vi "Teleop.vi"(10 "Match Info":T1={"Autonomous Elapsed Seconds"=0.0, "TeleOp Elapsed Seconds"=0.0, "Disabled Elapsed Seconds"=0.0, "Visited Autonomous"=FALSE, "Visited TeleOp"=FALSE, "Visited Disabled"=FALSE, "Autonomous Settings"={"Autonomous Style"=enum."Independent", "VI Refnum"=refnum}}, 11 "Call Context":T2) -> ()   [LabVIEW 2016]
doc: "This VI is called for each TeleOp packet received from the DS where the robot is not disabled. It is often used to read from the joysticks and update I/O or to update setpoints for timed control loops. It should complete and return within 20 milliseconds or it may miss DS packets."
uses:
  <vilib>/Rock Robotics/WPI/DriverStation/WPI_DriverStationDerivedRobotMode.ctl
  <vilib>/Rock Robotics/WPI/DriverStation/WPI_DriverStationMatch Info.ctl
  <vilib>/Rock Robotics/WPI/Solenoid/WPI_SolenoidValue.ctl
  <vilib>/Rock Robotics/WPI/ThirdParty/CanMotor/TalonSRX/WPI_CANTalonSRX_APIControlMode.ctl
  <vilib>/Rock Robotics/WPI/Relay/WPI_RelayValue.ctl
  <vilib>/Rock Robotics/WPI/Utilities/WPI_GetSetVariantRefNum.vi
  <vilib>/Rock Robotics/Network Tables/NT Write Boolean Array.vi
  <vilib>/Rock Robotics/Network Tables/NT Write Numeric Array.vi
  <vilib>/Rock Robotics/Network Tables/NT Read Boolean.vi
  <vilib>/Rock Robotics/Network Tables/NT Read Number.vi
  Robot Global Data.vi
  <vilib>/Rock Robotics/WPI/Solenoid/WPI_SolenoidSetEnum.vi
panel:
  out "Sensor":dbl(graph)
  in  "reset angle":bool
  out "shifter toggle":dbl
  out "Angle":dbl
  out "Numeric 2":dbl
  out "Numeric":dbl
  in  "invert?":bool
  in  "intput":bool
  out "Sample Slider 0":dbl(slide) scale=0.0..5.0
  out "Sample Boolean 1":bool
  out "Sample Boolean 0":bool
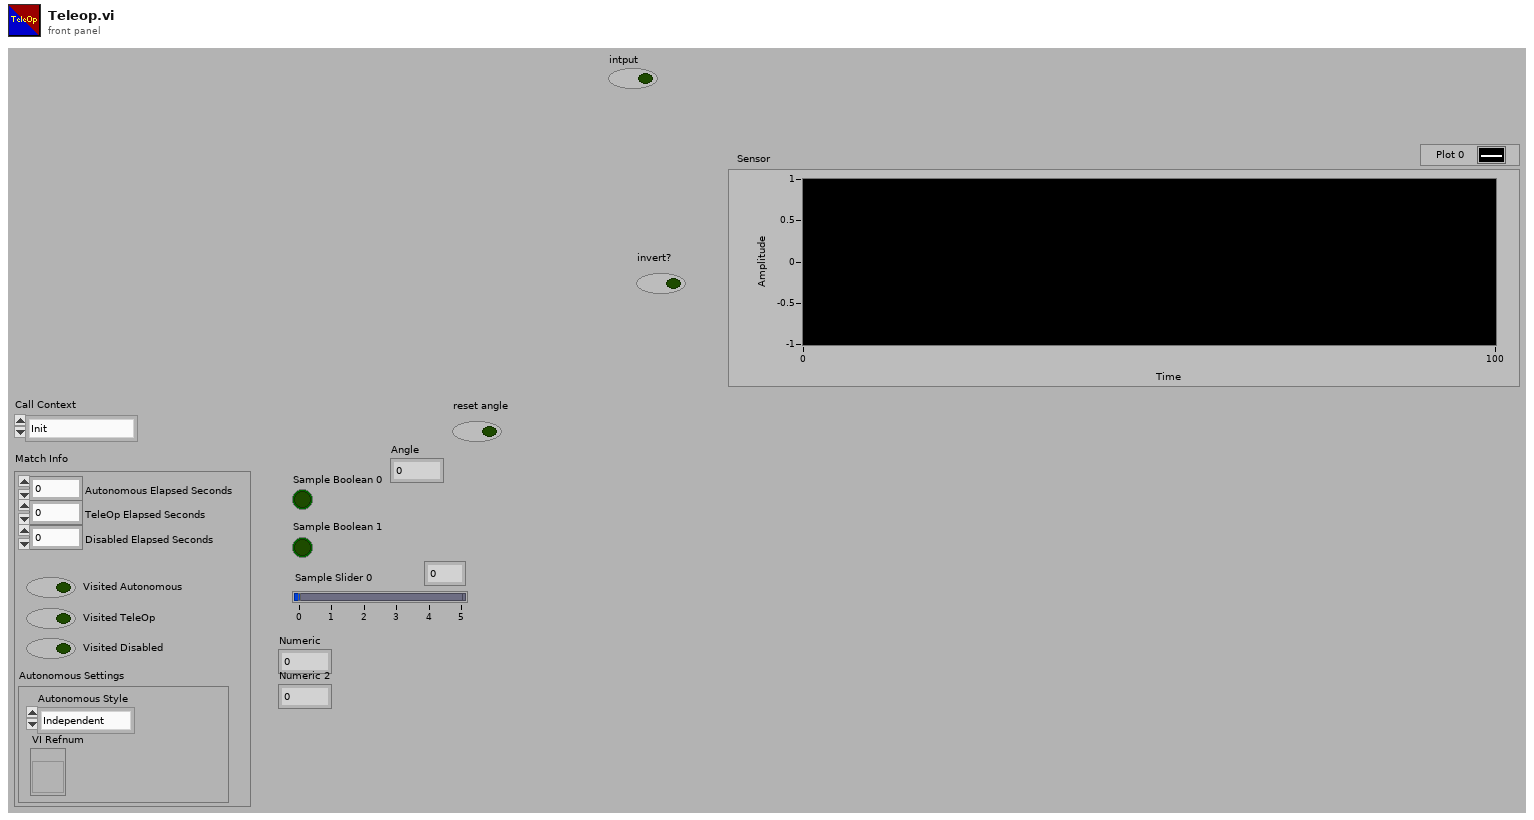
[diagram p1: front panel]
types:
  T1 = typedef "WPI_DriverStationMatch Info.ctl" = cluster{"Autonomous Elapsed Seconds":dbl, "TeleOp Elapsed Seconds":dbl, "Disabled Elapsed Seconds":dbl, "Visited Autonomous":bool, "Visited TeleOp":bool, "Visited Disabled":bool, "Autonomous Settings":cluster{"Autonomous Style":enum16{"Iterative", "Independent"}, "VI Refnum":refnum<vi>}}
  T2 = typedef "WPI_DriverStationDerivedRobotMode.ctl" = enum16{"Init", "Execute", "Stop"}
  T3 = typedef "WPI_SolenoidValue.ctl" = enum16{"Off", "On", "Forward", "Reverse"}
  T4 = typedef "WPI_GyroDevRef.ctl" = cluster{"DevStatus":errorcluster, "Analog Channel":T5, "Offset":dbl, "Gain (VoltsPerDegree/Second)":dbl, "Gyro Type":enum16{"Analog", "XRS450"}, "Handle":i32, "SPI Bus":T6, "Device Found":bool, "Sample Rate":dbl, "Calibrate On Open":bool}
  T5 = typedef "FPGA_AIChannel.ctl" = enum8{"AI 0", "AI 1", "AI 2", "AI 3", "AI MXP 0", "AI MXP 1", "AI MXP 2", "AI MXP 3", "Invalid"}
  T6 = typedef "spi_bus.ctl" = enum16{"SPI On-Board, CS0", "SPI On-Board, CS1", "SPI On-Board, CS2", "SPI On-Board, CS3", "SPI MXP", "Invalid"}
  T7 = typedef "WPI_EncoderDevRef.ctl" = cluster{"DevStatus":errorcluster, "EncoderIndex":T8, "CounterIndex":T9, "DistancePerCount":dbl, "Decoding Type":T10}
  T8 = typedef "FPGA_EncoderIdx.ctl" = enum8{"Enc 0", "Enc 1", "Enc 2", "Enc 3", "Enc 4", "Enc 5", "Enc 6", "Enc 7", "Invalid"}
  T9 = typedef "FPGA_CounterCtrSystemIndex.ctl" = enum8{"Ctr 0", "Ctr 1", "Ctr 2", "Ctr 3", "Ctr 4", "Ctr 5", "Ctr 6", "Ctr 7", "Invalid"}
  T10 = typedef "WPI_EncoderType.ctl" = enum16{"1x", "2x", "4x"}
  T11 = typedef "WPI_JoystickDevRef.ctl" = cluster{"Device":T12}
  T12 = typedef "WPI_JoystickDeviceEnum.ctl" = enum16{"USB 0", "USB 1", "USB 2", "USB 3", "USB 4", "USB 5"}
  T13 = typedef "WPI_SolenoidDevRef.ctl" = cluster{"DevStatus":errorcluster, "Pneumatics Control Module":u8, "Forward Solenoid Channel":T14, "Reverse Solenoid Channel":T14}
  T14 = typedef "WPI_SolenoidChannel.ctl" = enum8{"Solenoid 0", "Solenoid 1", "Solenoid 2", "Solenoid 3", "Solenoid 4", "Solenoid 5", "Solenoid 6", "Solenoid 7", "Invalid"}
  T15 = typedef "WPI_MotorControlDeviceRef.ctl" = cluster{"DeviceStatus":errorcluster, "Type":T16, "PWM":cluster{"PWM Channel":T17, "DeadBand":T18}, "CAN":cluster{"Device Number":u8, "SetOutput VI Ref":variant, "GetOutput VI Ref":variant, "Enable VI Ref":variant, "Disable VI Ref":variant, "Data":variant}, "Invert":bool}
  T16 = typedef "WPI_MotorControlType.ctl" = enum16{"PWM", "CAN"}
  T17 = typedef "FPGA_DIOPWMChannel.ctl" = enum8{"PWM 0", "PWM 1", "PWM 2", "PWM 3", "PWM 4", "PWM 5", "PWM 6", "PWM 7", "PWM 8", "PWM 9", "PWM MXP 0", "PWM MXP 1", "PWM MXP 2", "PWM MXP 3", "PWM MXP 4", "PWM MXP 5", "PWM MXP 6", "PWM MXP 7", "PWM MXP 8", "PWM MXP 9", "Invalid"}
  T18 = typedef "WPI_PWMDeadband.ctl" = cluster{"Name":string, "maxPositivePwm":i32, "minPositivePwm":i32, "centerPwm":i32, "maxNegativePwm":i32, "minNegativePwm":i32, "angularRange":u16}
  T19 = typedef "WPI_RobotDriveDevRef.ctl" = cluster{"DevStatus":errorcluster, "Motors[]":T15[], "Square Inputs":bool, "Max Output":dbl}
  T20 = typedef "WPI_CANTalonSRX_APIControlMode.ctl" = enum8{"Percent VBus", "Speed", "Position", "Slave", "Unchanged / Invalid", "Voltage Compensation", "Current", "Motion Profile", "Motion Magic"}
  T21 = typedef "WPI_RelayValue.ctl" = enum16{"Off", "On", "Forward", "Reverse"}
  T22 = typedef "WPI_CANTalonSRX_GlobalStatus.ctl" = cluster{"Applied Throttle":dbl, "Module Enabled":bool, "CAN Error":errorcluster, "Closed Loop Error":dbl, "Forward Limit Switch Closed":bool, "Reverse Limit Switch Closed":bool, "Sensor Position":dbl, "Sensor Velocity":dbl, "Current":dbl, "Sticky Fault - Over Temp":bool, "Sticky Fault - Under Voltage":bool, "Sticky Fault - Forward Limit":bool, "Sticky Fault - Reverse Limit":bool, "Sticky Fault - Forward Soft Limit":bool, "Sticky Fault - Reverse Soft Limit":bool, "Brake is Enabled":bool, "Encoder Position":dbl, "Encoder Velocity":dbl, "Encoder Index Count":dbl, "Encoder A Pin State":bool, "Encoder B Pin State":bool, "Encoder Index Pin State":bool, "Analog In":dbl, "Analog In Velocity":dbl, "Temperature (C)":dbl, "Battery Voltage":dbl, "Control 5 Is Supported":bool, "Current Profile Slot Select":dbl, "Pos Div 8":bool, "Vel Div 4":bool, "Pulse Width Position":i32, "Pulse Width Velocity":i32, "Pulse Width Rise To Rise (us)":i32, "Pulse Width Rise To Fall (us)":i32, "Mot Prof Active Is Under Run":bool, "Mot Prof Active Has Under Run":bool, "Mot Prof Active Is Last":bool, "Mot Prof Active Velocity Only":bool, "Mot Prof Active Is Valid":bool, "Mot Prof Buffer Is Full":bool, "Mot Prof Active Profile Slot Select":i32, "Mot Prof NextID":i32, "Mot Prof Count":i32, "Mot Prof Active Velocity":dbl, "Mot Prof Active Position":dbl, "Mot Prof Output Enable":i32}
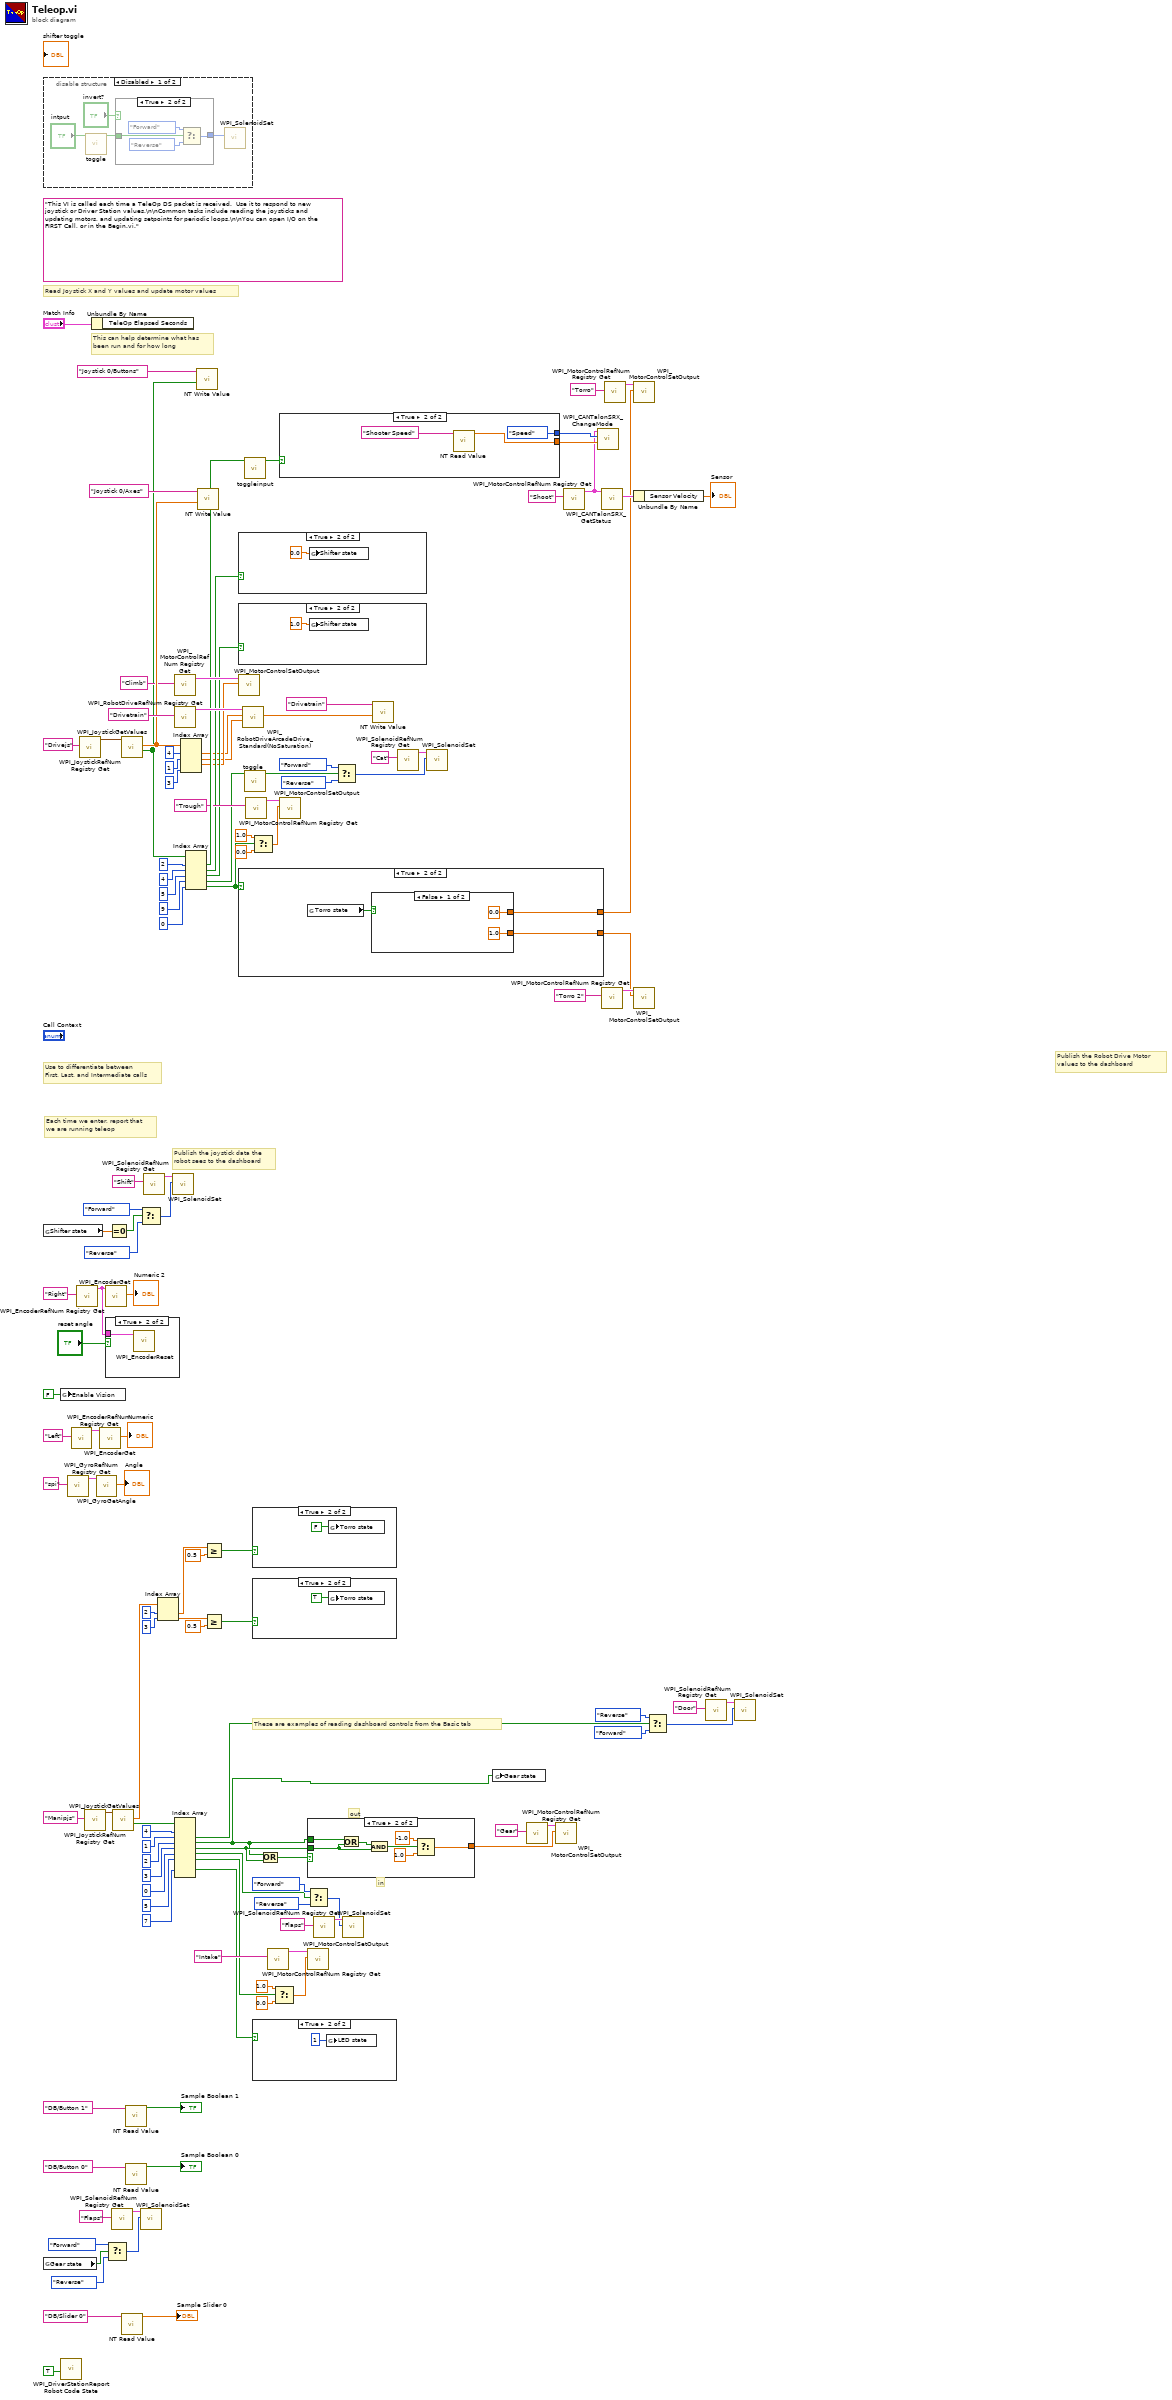
[diagram p0: block diagram]
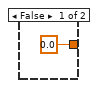
[diagram p2: hidden frame]
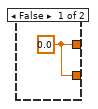
[diagram p3: hidden frame]
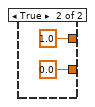
[diagram p4: hidden frame]
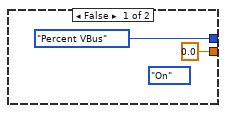
[diagram p7: hidden frame]
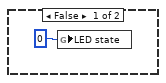
[diagram p9: hidden frame]
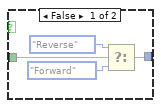
[diagram p12: hidden frame]
diagram:
  (unwired) "This VI is called each time a TeleOp DS packet is received.  Use it to respond to new joystick or Driver Station values.\n\nCommon tasks include reading the joysticks and updating motors, and updating setpoints for periodic loops.\n\nYou can open I/O on the FIRST Call, or in the Begin.vi."
  # "out"
  # "in"
  # "These are examples of reading dashboard controls from the Basic tab"
  # "Publish the Robot Drive Motor\nvalues to the dashboard"
  # "Publish the joystick data the\nrobot sees to the dashboard"
  # "Each time we enter, report that\nwe are running teleop"
  # "Use to differentiate between\nFirst, Last, and Intermediate calls"
  # "This can help determine what has\nbeen run and for how long"
  # "Read Joystick X and Y values and update motor values"
  n1 = disable-structure shown="Disabled" {
    frame Disabled {
      n2 = call "toggle.vi"("Boolean"="intput") -> ("Boolean 2"=w130:bool)  [unwired: 10 in]
      n3 = case shown="True" "invert?" {
        tunnel: [w135 w138] -> w129
        tunnel: w130 -> [w133 w137]
        frame False {
          n4 = Select(t=WPI_SolenoidValue."Reverse" ("Value"), s=w133, f=WPI_SolenoidValue."Forward" ("Value")) -> (s? t:f=w135:T3)
        }
        frame True {
          n5 = Select(t=WPI_SolenoidValue."Forward" ("Value"), s=w137, f=WPI_SolenoidValue."Reverse" ("Value")) -> (s? t:f=w138:T3)
        }
      }
      n6 = call-poly <vilib>:"WPI_SolenoidSet.vi"("Value"=w129) -> ()  [unwired: 9 in, 2 out]
    }
    frame Enabled {
    }
  }
  n7 = global read "Robot Global Data.vi" "Shifter state"() -> (w64:dbl)
  n8 = global read "Robot Global Data.vi" "Gear state"() -> (w7:bool)
  n9 = global write "Robot Global Data.vi" "Enable Vision"(FALSE ("Enable Vision")) -> ()
  n10 = call <vilib>:"WPI_DriverStationReport Robot Code State.vi"("TeleOp"=TRUE ("Autonomous")) -> ()  [unwired: 10 in, 1 out]
  n11 = call <vilib>:"WPI_GyroRefNum Registry Get.vi"("refnum name"="spi") -> ("GyroDevRef"=w52:T4)  [unwired: 9 in, 1 out]
  n12 = call <vilib>:"WPI_EncoderRefNum Registry Get.vi"("refnum name"="Left") -> ("EncoderDevRef"=w95:T7)  [unwired: 9 in, 1 out]
  n13 = call <vilib>:"WPI_EncoderRefNum Registry Get.vi"("refnum name"="Right") -> ("EncoderDevRef"=w51:T7)  [unwired: 9 in, 1 out]
  n14 = call <vilib>:"WPI_JoystickRefNum Registry Get.vi"("refnum name"="Drivejs") -> ("JoystickDevRef"=w124:T11)  [unwired: 1 in, 9 out]
  n15 = call <vilib>:"WPI_JoystickRefNum Registry Get.vi"("refnum name"="Manipjs") -> ("JoystickDevRef"=w91:T11)  [unwired: 1 in, 9 out]
  n16 = Unbundle By Name("Match Info") -> ()  [unwired: 1 out]
  n17 = call <vilib>:"WPI_GyroGetAngle.vi"("GyroDevRef"=w52) -> ("Angle"=→"Angle":dbl)  [unwired: 6 in, 4 out]
  n18 = call <vilib>:"WPI_EncoderGet.vi"("EncoderDevRef"=w95) -> ("Distance"=→"Numeric":dbl)  [unwired: 5 in, 5 out]
  n19 = call <vilib>:"WPI_EncoderGet.vi"("EncoderDevRef"=w51) -> ("Distance"=→"Numeric 2":dbl)  [unwired: 5 in, 5 out]
  n20 = case shown="True" "reset angle" {
    tunnel: w51 -> [_ w141]
    frame False {
    }
    frame True {
      n21 = call <vilib>:"WPI_EncoderReset.vi"("EncoderDevRef"=w141) -> ()  [unwired: 9 in, 2 out]
    }
  }
  n22 = Select(t=WPI_SolenoidValue."Forward" ("Value"), s=w7, f=WPI_SolenoidValue."Reverse" ("Value")) -> (s? t:f=w8:T3)
  n23 = Equal To 0?(x=w64) -> (x = 0?=w65:bool)
  n24 = call <vilib>:"WPI_SolenoidRefNum Registry Get.vi"("refnum name"="Flaps") -> ("SolenoidDevRef"=w11:T13)  [unwired: 9 in, 1 out]
  n25 = call <vilib>:"WPI_JoystickGetValues.vi"("JoystickDevRef"=w91) -> ("Buttons"=w90:bool[], "Axes"=w44:dbl[])  [unwired: 6 in, 3 out]
  n26 = call <vilib>:"WPI_JoystickGetValues.vi"("JoystickDevRef"=w124) -> ("Buttons"=w89:bool[], "Axes"=w120:dbl[])  [unwired: 6 in, 3 out]
  n27 = call-poly <vilib>:"NT Read Value.vi"("Name"="DB/Slider 0" ("refnum name")) -> ("Numeric"=→"Sample Slider 0":dbl)  [unwired: 9 in, 1 out]
  n28 = call-poly <vilib>:"NT Read Value.vi"("Name"="DB/Button 1" ("refnum name")) -> ("Boolean"=→"Sample Boolean 1":bool)  [unwired: 9 in, 1 out]
  n29 = call-poly <vilib>:"NT Read Value.vi"("Name"="DB/Button 0" ("refnum name")) -> ("Boolean"=→"Sample Boolean 0":bool)  [unwired: 9 in, 1 out]
  n30 = Select(t=WPI_SolenoidValue."Forward" ("Value"), s=w65, f=WPI_SolenoidValue."Reverse" ("Value")) -> (s? t:f=w73:T3)
  n31 = call-poly <vilib>:"WPI_SolenoidSet.vi"("Value"=w8, "SolenoidDevRef"=w11) -> ()  [unwired: 8 in, 2 out]
  n32 = call <vilib>:"WPI_SolenoidRefNum Registry Get.vi"("refnum name"="Shift") -> ("SolenoidDevRef"=w72:T13)  [unwired: 9 in, 1 out]
  n33 = Index Array(array=w44, index #1=2 ("index"), index #2=3 ("index")) -> (element #1=w40:dbl, element #2=w38:dbl)
  n34 = call-poly <vilib>:"WPI_SolenoidSet.vi"("Value"=w73, "SolenoidDevRef"=w72) -> ()  [unwired: 8 in, 2 out]
  n35 = call <vilib>:"WPI_MotorControlRefNum Registry Get.vi"("refnum name"="Climb") -> ("MotorControlDevRef"=w108:T15)  [unwired: 9 in, 1 out]
  n36 = call <vilib>:"WPI_RobotDriveRefNum Registry Get.vi"("refnum name"="Drivetrain") -> ("RobotDriveDevRef"=w126:T19)  [unwired: 1 in, 9 out]
  n37 = Index Array(array=w90, index #1=4 ("index"), index #2=1 ("index"), index #3=2 ("index"), index #4=3 ("index"), index #5=0 ("index"), index #6=5 ("index"), index #8=7 ("index")) -> (element #2=w26:bool, element #3=w1:bool, element #4=w3:bool, element #5=w27:bool, element #6=w60:bool, element #8=w54:bool)  [unwired: 2 in, 3 out]
  n38 = Index Array(array=w120, index #1=4 ("index"), index #2=1 ("index"), index #4=3 ("index")) -> (element #1=w24:dbl, element #2=w23:dbl, element #3=w59:dbl)  [unwired: 1 in, 1 out]
  n39 = Index Array(array=w89, index #1=2 ("index"), index #2=4 ("index"), index #3=5 ("index"), index #4=9 ("index"), index #5=0 ("index")) -> (element #1=w86:bool, element #2=w67:bool, element #3=w66:bool, element #4=w21:bool, element #5=w30:bool)
  n40 = call-poly <vilib>:"NT Write Value.vi"("Boolean Array"=w89, "Name"="Joystick 0/Buttons") -> ()  [unwired: 9 in, 1 out]
  n41 = call-poly <vilib>:"NT Write Value.vi"("Numeric Array"=w120, "Name"="Joystick 0/Axes") -> ()  [unwired: 9 in, 1 out]
  n42 = Greater Or Equal?(x=w40, y=0.5) -> (x >= y?=w39:bool)
  n43 = Greater Or Equal?(x=w38, y=0.5) -> (x >= y?=w36:bool)
  n44 = case shown="True" w67 {
    frame False {
    }
    frame True {
      n45 = global write "Robot Global Data.vi" "Shifter state"(0.0 ("shifter toggle")) -> ()
    }
  }
  n46 = case shown="True" w66 {
    frame False {
    }
    frame True {
      n47 = global write "Robot Global Data.vi" "Shifter state"(1.0 ("shifter toggle")) -> ()
    }
  }
  n48 = call <vilib>:"WPI_MotorControlSetOutput.vi"("Output"=w59, "MotorControlDevRef"=w108) -> ()  [unwired: 7 in, 3 out]
  n49 = case shown="True" w30 {
    tunnel: [w144 w146] -> w29
    tunnel: [w144 w145] -> w28
    frame False {
      w144 = 0.0 ("Output")
    }
    frame True {
      n50 = global read "Robot Global Data.vi" "Torro state"() -> (w147:bool)
      n51 = case shown="False" w147 {
        tunnel: [0.0 ("Output") 1.0 ("Output")] -> w146
        tunnel: [1.0 ("Output") 0.0 ("Output")] -> w145
        frame False {
        }
        frame True {
        }
      }
    }
  }
  n52 = call <vilib>:"WPI_RobotDriveArcadeDrive_Standard(NoSaturation).vi"("Y axis value"=w23, "X axis value"=w24, "RobotDriveDevRef"=w126) -> ("Motor Values"=w113:dbl[])  [unwired: 1 in, 7 out]
  n53 = call "toggleinput.vi"("Boolean"=w86) -> ("Boolean 2"=w35:bool)  [unwired: 10 in]
  n54 = call "toggle.vi"("Boolean"=w21) -> ("Boolean 2"=w15:bool)  [unwired: 10 in]
  n55 = call <vilib>:"WPI_MotorControlRefNum Registry Get.vi"("refnum name"="Trough") -> ("MotorControlDevRef"=w84:T15)  [unwired: 9 in, 1 out]
  n56 = Select(t=1.0, s=w30, f=0.0) -> (s? t:f=w31:dbl)
  n57 = case shown="True" w39 {
    frame False {
    }
    frame True {
      n58 = global write "Robot Global Data.vi" "Torro state"(FALSE ("Torro state")) -> ()
    }
  }
  n59 = case shown="True" w36 {
    frame False {
    }
    frame True {
      n60 = global write "Robot Global Data.vi" "Torro state"(TRUE ("Torro state")) -> ()
    }
  }
  n61 = case shown="True" w54 {
    frame False {
      n62 = global write "Robot Global Data.vi" "LED state"(i8 0 ("LED state")) -> ()
    }
    frame True {
      n63 = global write "Robot Global Data.vi" "LED state"(i8 1 ("LED state")) -> ()
    }
  }
  n64 = Or(x=w1, y=w3) -> (x .or. y?=w4:bool)
  n65 = call <vilib>:"WPI_MotorControlRefNum Registry Get.vi"("refnum name"="Intake") -> ("MotorControlDevRef"=w79:T15)  [unwired: 9 in, 1 out]
  n66 = Select(t=1.0, s=w60, f=0.0) -> (s? t:f=w78:dbl)
  n67 = case shown="True" w35 {
    tunnel: [WPI_CANTalonSRX_APIControlMode."Percent VBus" ("Control Mode") WPI_CANTalonSRX_APIControlMode."Speed" ("Control Mode")] -> w46
    tunnel: [0.0 ("Numeric") w158] -> w45
    frame False {
      (unwired) WPI_RelayValue."On" ("RelayValue")
    }
    frame True {
      n68 = call-poly <vilib>:"NT Read Value.vi"("Name"="Shooter Speed") -> ("Numeric"=w158:dbl)  [unwired: 9 in, 1 out]
    }
  }
  n69 = call <vilib>:"WPI_MotorControlSetOutput.vi"("Output"=w31, "MotorControlDevRef"=w84) -> ()  [unwired: 7 in, 3 out]
  n70 = case shown="True" w4 {
    tunnel: w3 -> [_ w166]
    tunnel: w1 -> [_ w168]
    tunnel: [0.0 w162] -> w2
    frame False {
    }
    frame True {
      n71 = Or(x=w168, y=w166) -> (x .or. y?=w167:bool)
      n72 = And(x=w167, y=w166) -> (x .and. y?=w165:bool)
      n73 = Select(t=-1.0, s=w165, f=1.0) -> (s? t:f=w162:dbl)
    }
  }
  n74 = call <vilib>:"WPI_MotorControlSetOutput.vi"("Output"=w78, "MotorControlDevRef"=w79) -> ()  [unwired: 7 in, 3 out]
  n75 = Select(t=WPI_SolenoidValue."Forward" ("Value"), s=w27, f=WPI_SolenoidValue."Reverse" ("Value")) -> (s? t:f=w99:T3)
  n76 = call <vilib>:"WPI_SolenoidRefNum Registry Get.vi"("refnum name"="Flaps") -> ("SolenoidDevRef"=w101:T13)  [unwired: 9 in, 1 out]
  n77 = Select(t=WPI_SolenoidValue."Forward" ("Value"), s=w15, f=WPI_SolenoidValue."Reverse" ("Value")) -> (s? t:f=w18:T3)
  n78 = call-poly <vilib>:"WPI_SolenoidSet.vi"("Value"=w99, "SolenoidDevRef"=w101) -> ()  [unwired: 8 in, 2 out]
  n79 = call-poly <vilib>:"NT Write Value.vi"("Numeric Array"=w113, "Name"="Drivetrain") -> ()  [unwired: 9 in, 1 out]
  n80 = call <vilib>:"WPI_SolenoidRefNum Registry Get.vi"("refnum name"="Cat") -> ("SolenoidDevRef"=w17:T13)  [unwired: 9 in, 1 out]
  n81 = call-poly <vilib>:"WPI_SolenoidSet.vi"("Value"=w18, "SolenoidDevRef"=w17) -> ()  [unwired: 8 in, 2 out]
  n82 = global write "Robot Global Data.vi" "Gear state"(w1) -> ()
  n83 = call <vilib>:"WPI_MotorControlRefNum Registry Get.vi"("refnum name"="Gear") -> ("MotorControlDevRef"=w5:T15)  [unwired: 9 in, 1 out]
  n84 = call <vilib>:"WPI_MotorControlSetOutput.vi"("Output"=w2, "MotorControlDevRef"=w5) -> ()  [unwired: 7 in, 3 out]
  n85 = call <vilib>:"WPI_MotorControlRefNum Registry Get.vi"("refnum name"="Shoot") -> ("MotorControlDevRef"=w25:T15)  [unwired: 9 in, 1 out]
  n86 = call <vilib>:"WPI_CANTalonSRX_ChangeMode.vi"("Output"=w45, "Control Mode"=w46, "CAN Talon SRX Ref"=w25) -> ()  [unwired: 7 in, 2 out]
  n87 = call <vilib>:"WPI_CANTalonSRX_GetStatus.vi"("CAN Talon SRX Ref"=w25) -> ("Talon SRX Status"=w49:T22)  [unwired: 8 in, 2 out]
  n88 = call <vilib>:"WPI_MotorControlRefNum Registry Get.vi"("refnum name"="Torro 2") -> ("MotorControlDevRef"=w47:T15)  [unwired: 9 in, 1 out]
  n89 = call <vilib>:"WPI_MotorControlRefNum Registry Get.vi"("refnum name"="Torro") -> ("MotorControlDevRef"=w32:T15)  [unwired: 9 in, 1 out]
  n90 = call <vilib>:"WPI_MotorControlSetOutput.vi"("Output"=w29, "MotorControlDevRef"=w32) -> ()  [unwired: 7 in, 3 out]
  n91 = Unbundle By Name(w49) -> ("Sensor Velocity"=→"Sensor":dbl)
  n92 = call <vilib>:"WPI_MotorControlSetOutput.vi"("Output"=w28, "MotorControlDevRef"=w47) -> ()  [unwired: 7 in, 3 out]
  n93 = Select(t=WPI_SolenoidValue."Reverse" ("Value"), s=w26, f=WPI_SolenoidValue."Forward" ("Value")) -> (s? t:f=w104:T3)
  n94 = call <vilib>:"WPI_SolenoidRefNum Registry Get.vi"("refnum name"="Door") -> ("SolenoidDevRef"=w106:T13)  [unwired: 9 in, 1 out]
  n95 = call-poly <vilib>:"WPI_SolenoidSet.vi"("Value"=w104, "SolenoidDevRef"=w106) -> ()  [unwired: 8 in, 2 out]
